vi "Discovery.vi"() -> (0 "error out":errorcluster, 3 "IP":string)   [LabVIEW 2016]
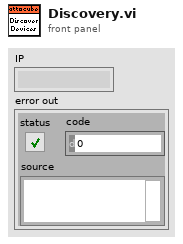
[diagram p1: front panel]
types:
  T1 = cluster{"IP":string, "DeviceType":string, "SerialNumber":string, "DeviceName":string, "macAddress":string, "locked":bool}[]
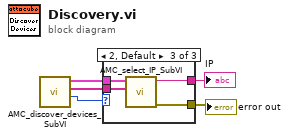
[diagram p0: block diagram]
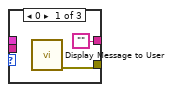
[diagram p2: hidden frame]
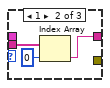
[diagram p3: hidden frame]
diagram:
  n1 = call "AMC_discover_devices_SubVI.vi"() -> ("No. of found devices"=w3:i32, "IPs"=w4:string[], "Found Devices"=w5:T1)  [unwired: 8 in, 1 out]
  n2 = case shown="2, Default" w3 {
    tunnel: w5 -> [_ _ w14]
    tunnel: w4 -> [_ w9 w13]
    tunnel: ["" w8 w12] -> w2
    tunnel: [w6 _ w11] -> w1
    frame 0 {
      n3 = call "Display Message to User"() -> ("error out"=w6:errorcluster)  [unwired: 10 in, 1 out]
    }
    frame 1 {
      n4 = Index Array(array=w9, index=0) -> (element=w8:string)
    }
    frame 2, Default {
      n5 = call "AMC_select_IP_SubVI.vi"("IPs"=w13, "Found Devices"=w14) -> ("error out"=w11:errorcluster, "IP"=w12:string)  [unwired: 7 in, 1 out]
    }
  }
  "IP" <- w2
  "error out" <- w1
